vi "Autonomous Independent.vi"() -> ()   [LabVIEW 2011]
doc: "This VI is called when autonomous begins, and will automatically be terminated when autonomous ends. You can carry out timed or sensor driven robot movement independently without needing to return to the caller."
uses:
  <vilib>/Rock Robotics/WPI/Relay/WPI_RelayValue.ctl
  Robot Global Data.vi
  <vilib>/Rock Robotics/WPI/RobotDrive/WPI_RobotDriveArcadeDrive_Standard(NoSaturation).vi
  cupStateGlobal.vi
  InfoTransferGlobal.vi
  <vilib>/ptbypt/NI_PtbyPt.lvlib
panel:
  out "Fixed Distance[m]":dbl
  in  "Slide 3":dbl(slide) scale=400.0..2000.0
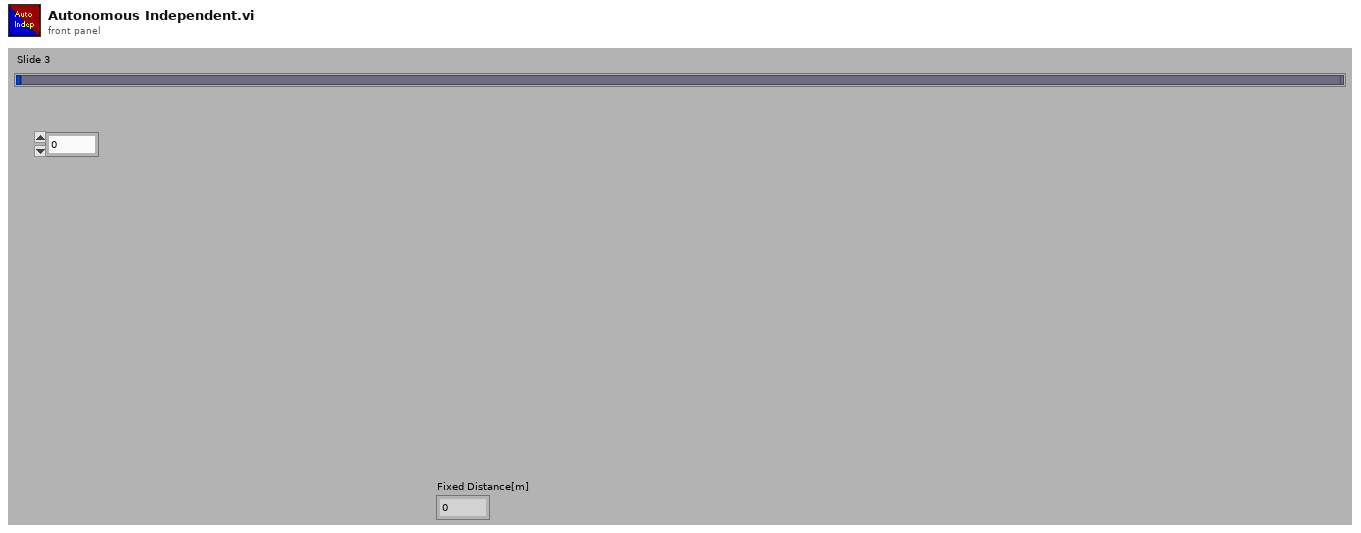
[diagram p1: front panel]
types:
  T1 = typedef "WPI_JoystickDevRef.ctl" = cluster{"Device":T2}
  T2 = typedef "WPI_JoystickDeviceEnum.ctl" = enum16{"USB 1", "USB 2", "USB 3", "USB 4", "Kinect 1", "Kinect 2"}
  T3 = typedef "WPI_DigitalInputDevRef.ctl" = cluster{"DevStatus":errorcluster, "DIO Channel":T4, "Digital Module":T5}
  T4 = typedef "FPGA_DIOChannel.ctl" = enum8{"DIO 1", "DIO 2", "DIO 3", "DIO 4", "DIO 5", "DIO 6", "DIO 7", "DIO 8", "DIO 9", "DIO 10", "DIO 11", "DIO 12", "DIO 13", "DIO 14", "Invalid"}
  T5 = typedef "FPGA_TypedefDigitalModule.ctl" = enum16{"Digital Module 1", "Digital Module 2"}
  T6 = typedef "WPI_RelayValue.ctl" = enum16{"Off", "On", "Forward", "Reverse"}
  T7 = typedef "WPI_RobotDriveDevRef.ctl" = cluster{"DevStatus":errorcluster, "Motors[]":T8[], "Square Inputs":bool, "Max Output":dbl, "Isochronous":bool}
  T8 = typedef "WPI_MotorControlDeviceRef.ctl" = cluster{"DeviceStatus":errorcluster, "Type":enum16{"PWM", "CAN"}, "PWM":cluster{"Digital Module":T5, "PWM Channel":T9, "DeadBand":T10}, "CAN":cluster{"Device Number":u8, "Control Mode":T11, "Semaphore":T12, "Max Vout":dbl}, "Invert":bool, "TransformRef":T13, "InvTransformRef":T13}
  T9 = typedef "FPGA_DIOPWMChannel.ctl" = enum8{"PWM 1", "PWM 2", "PWM 3", "PWM 4", "PWM 5", "PWM 6", "PWM 7", "PWM 8", "PWM 9", "PWM 10", "Invalid"}
  T10 = typedef "WPI_PWMDeadband.ctl" = cluster{"Name":string, "maxPositivePwm":i32, "minPositivePwm":i32, "centerPwm":i32, "maxNegativePwm":i32, "minNegativePwm":i32, "angularRange":u16}
  T11 = typedef "WPI_CANJaguar_ControlMode.ctl" = enum8{"Percent VBus", "Current", "Speed", "Position", "Voltage"}
  T12 = typedef "Semaphore RefNum" = refnum<k1>
  T13 = typedef "WPI_PWMTransform_ConPane.ctl" = refnum<vi>
  T14 = typedef "WPI_EncoderDevRef.ctl" = cluster{"DevStatus":errorcluster, "EncoderIndex":T15, "CounterIndex":T16, "DistancePerCount":dbl, "Decoding Type":T17}
  T15 = typedef "FPGA_EncoderIdx.ctl" = enum8{"Enc 0", "Enc 1", "Enc 2", "Enc 3", "Invalid"}
  T16 = typedef "FPGA_CounterCtrSystemIndex.ctl" = enum8{"Ctr 0", "Ctr 1", "Ctr 2", "Ctr 3", "Ctr 4", "Ctr 5", "Ctr 6", "Ctr 7", "Invalid"}
  T17 = typedef "WPI_EncoderType.ctl" = enum16{"1x", "2x", "4x"}
  T18 = cluster{"RightAxis":dbl, "LeftAxis":dbl, "RightHead":bool, "Left Head":bool, "Left Leg Out":bool, "Left Leg Forward":bool, "Left Leg Back":bool, "Right Leg Out":bool, "Right Leg Forward":bool, "Right Leg Back":bool}
  T19 = typedef "WPI_RelayDevRef.ctl" = cluster{"DevStatus":errorcluster, "Relay Channel":T20, "Digital Module":T5, "Relay Direction":T21}
  T20 = typedef "FPGA_DIORelayChannel.ctl" = enum8{"Relay 1", "Relay 2", "Relay 3", "Relay 4", "Relay 5", "Relay 6", "Relay 7", "Relay 8", "Invalid"}
  T21 = typedef "WPI_RelayDirection.ctl" = enum16{"Both directions", "Forward only", "Reverse only"}
  T22 = typedef "WPI_AnalogChannelDevRef.ctl" = cluster{"DevStatus":errorcluster, "Analog Module":T23, "Analog Channel":T24}
  T23 = typedef "FPGA_TypedefAnalogModule.ctl" = enum16{"Analog Module 1", "Analog Module 2"}
  T24 = typedef "FPGA_AIChannel.ctl" = enum8{"AI 1", "AI 2", "AI 3", "AI 4", "AI 5", "AI 6", "AI 7", "AI 8", "Invalid"}
  T25 = cluster{"Selected Target Info":cluster{"Position":cluster{"X":dbl, "Y":dbl}, "Distance (m)":dbl, "Target Found?":bool}, "output cluster":cluster{"BottomOR":i16, "CupOR":i16, "TopOR":i16, "FloorOR":i16}, "keys pressed":enum16{"0", "1", "2", "3", "4", "5", "6", "7", "8", "9", "A", "B", "C", "D", "E", "F", "G", "H", "I", "J", "K", "L", "M", "N", "O", "P", "Q", "R", "S", "T", "U", "V", "W", "X", "Y", "Z", "F1", "F2", "F3", "F4", "F5", "F6", "F7", "F8", "F9", "F10", "F11", "F12", "F13", "F14", "F15", "ADD", "BACK", "BACKSLASH", "CAPITAL", "COMMA", "DECIMAL", "DELETE", "DIVIDE", "DOWN", "END", "EQUALS", "ESCAPE", "GRAVE (`)", "HOME", "INSERT", "LBRACKET", "LCONTROL", "LEFT", "L ALT", "LSHIFT", "LWIN", "MINUS", "MULTIPLY", "NEXT", "NUMLOCK", "NUMPAD_0", "NUMPAD_1", "NUMPAD_2", "NUMPAD_3", "NUMPAD_4", "NUMPAD_5", "NUMPAD_6", "NUMPAD_7", "NUMPAD_8", "NUMPAD_9", "PAUSE", "PERIOD", "PRIOR (PG UP)", "RBRACKET", "RCONTROL", "RETURN", "RIGHT", "R ALT", "RSHIFT", "RWIN", "SCROLL", "SEMICOLON", "SLASH", "SPACE", "SUBTRACT", "TAB", "UP", "ENTER (num pad)", "' (quote)"}[]}
  T26 = cluster{"Position":cluster{"X":dbl, "Y":dbl}, "Distance (m)":dbl, "Target Found?":bool}
  T27 = typedef "WPI_ServoDeviceRef.ctl" = cluster{"DeviceStatus":errorcluster, "Digital Module":T5, "PWM Channel":T9, "DeadBand":T10}
  T28 = cluster{"axis 1 (x)":dbl, "axis 2 (y)":dbl, "axis 3 (throttle)":dbl, "axis 4":dbl, "axis 5":dbl, "axis 6":dbl}
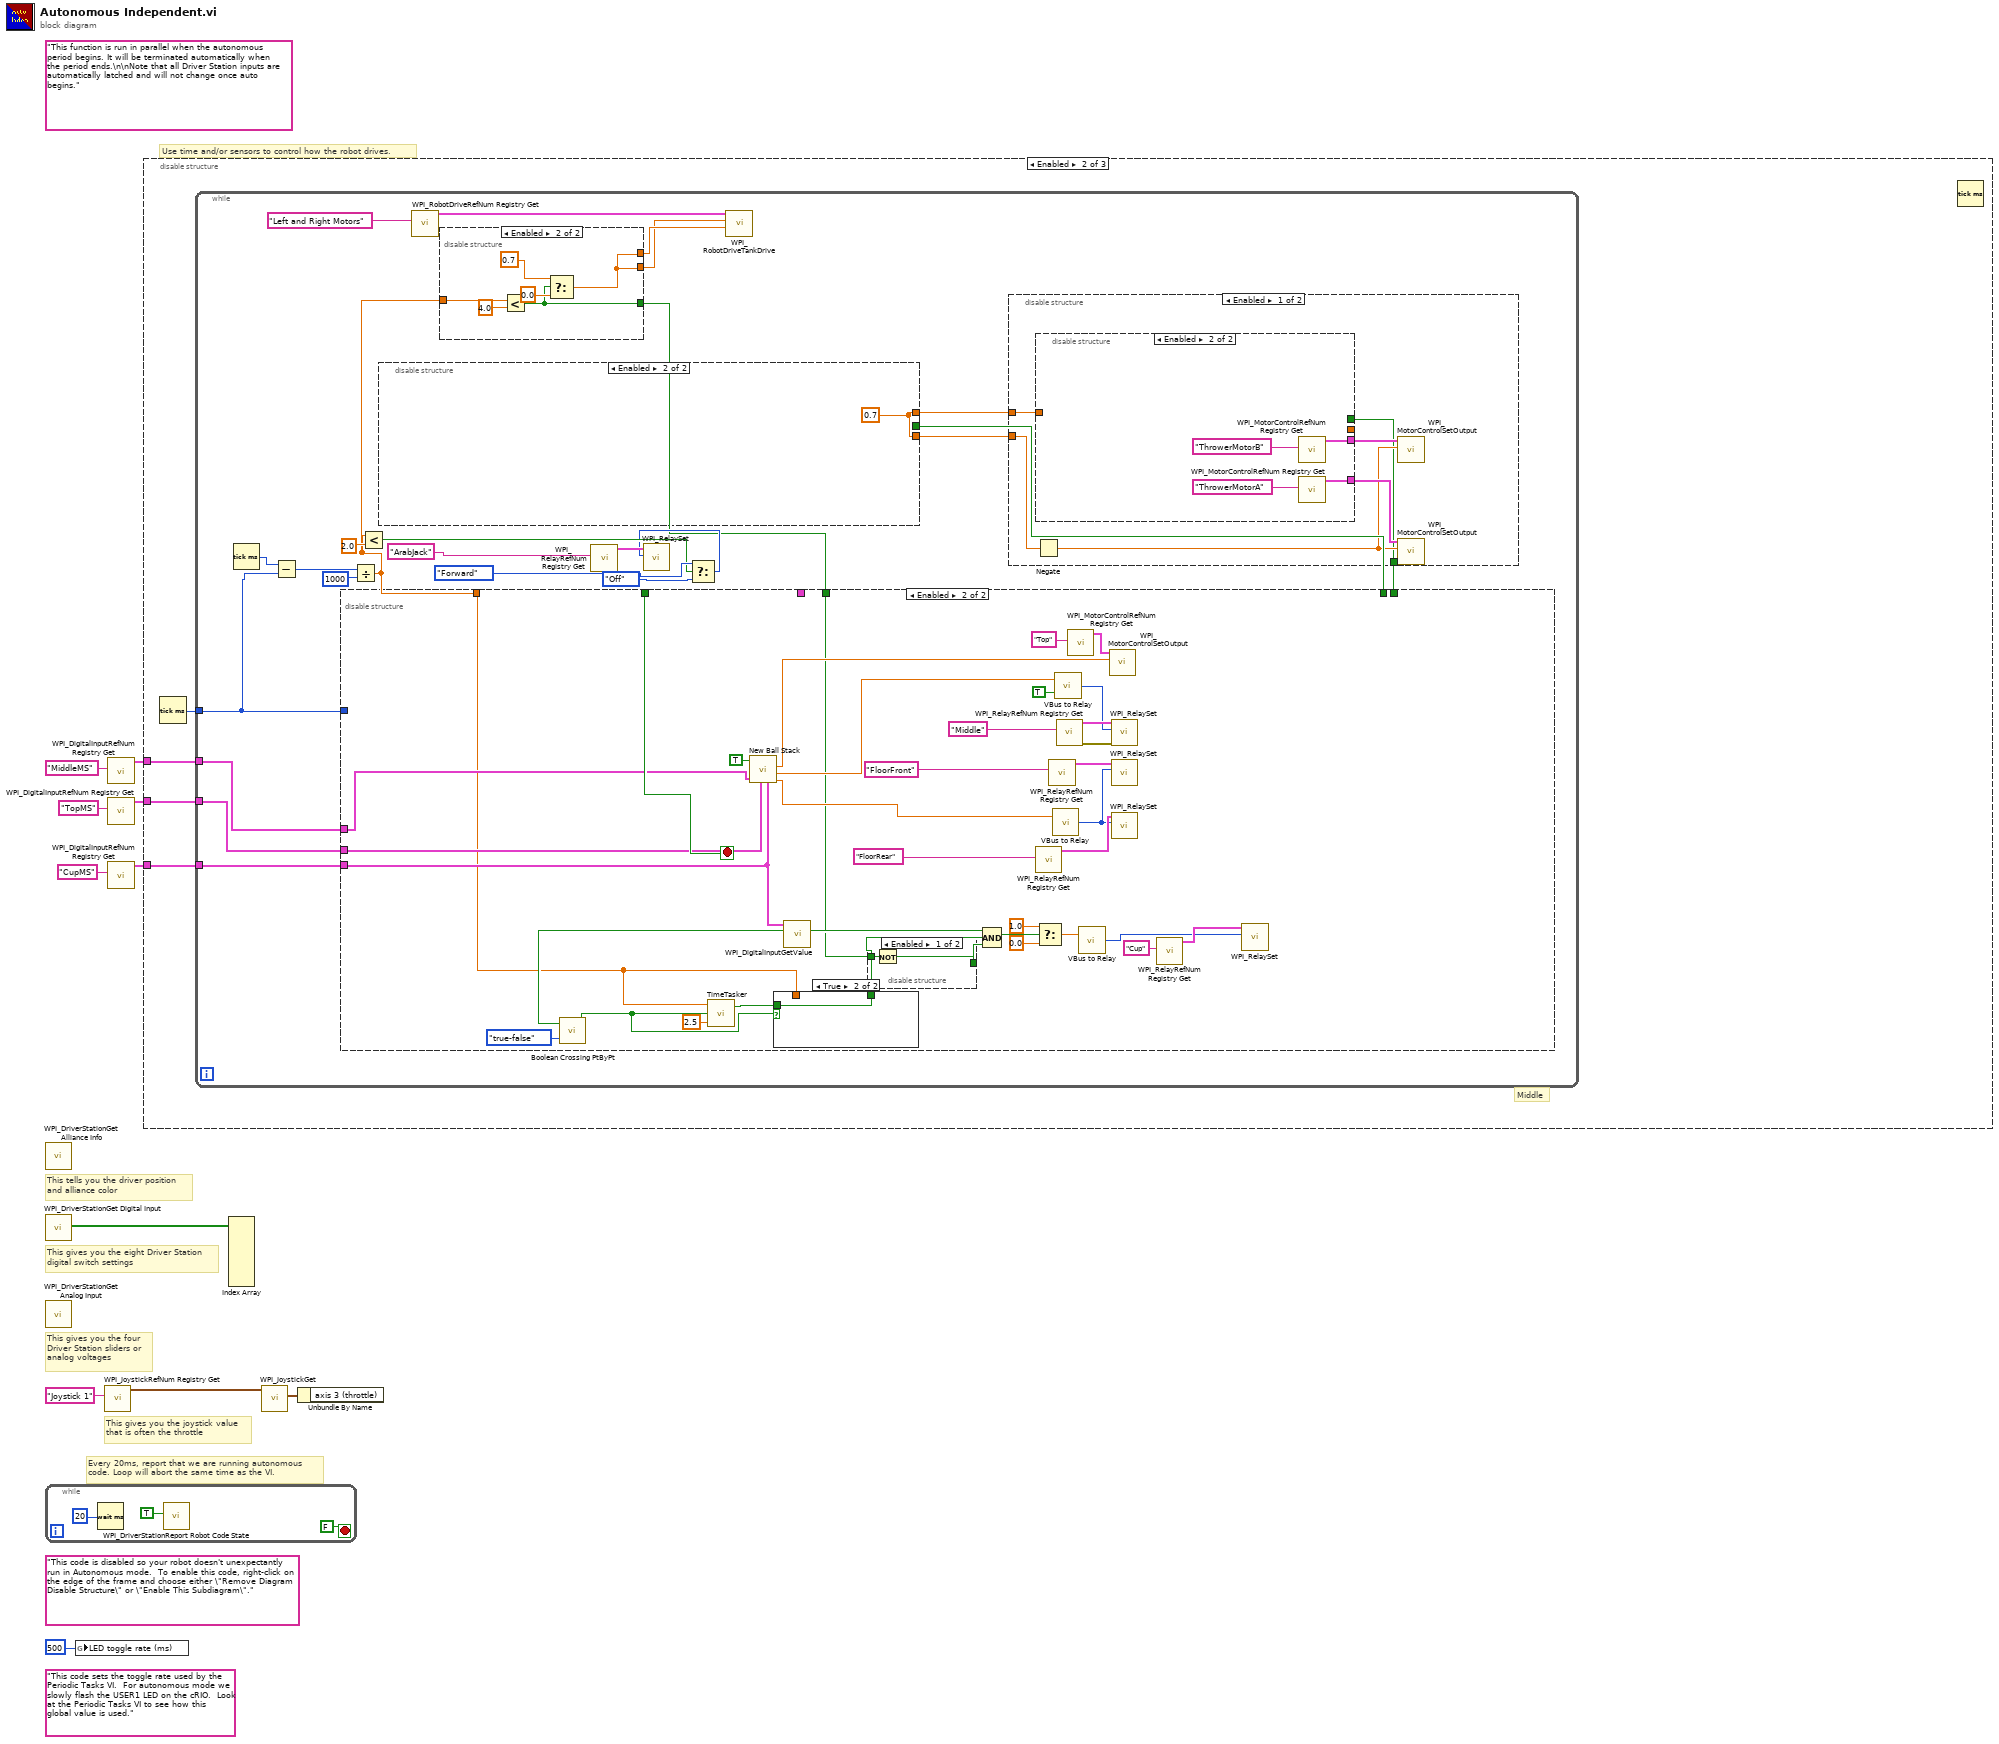
[diagram p0: block diagram]
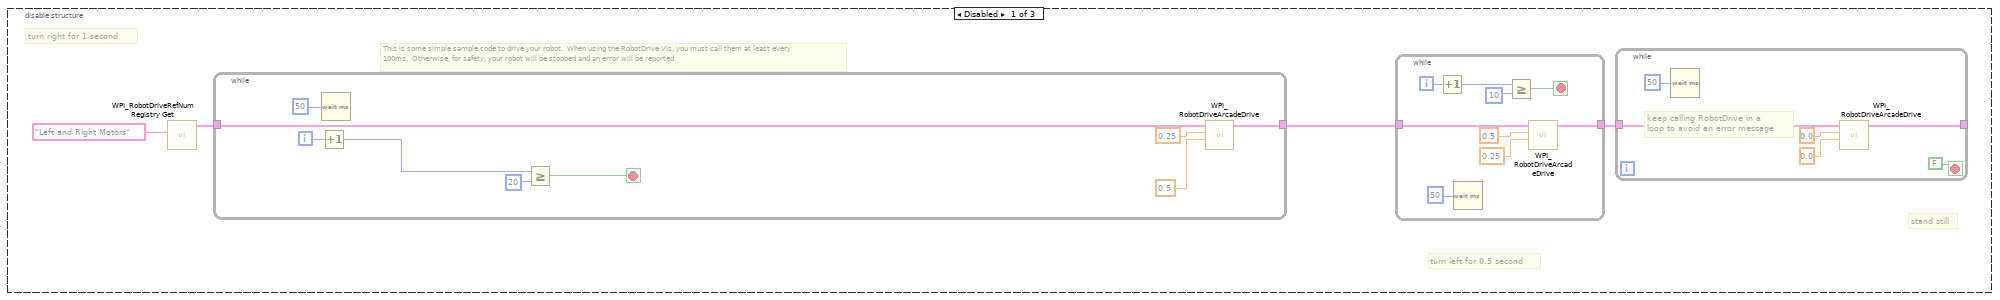
[diagram p2: hidden frame]
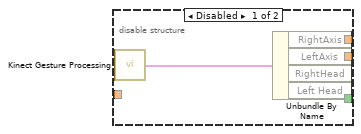
[diagram p3: hidden frame]
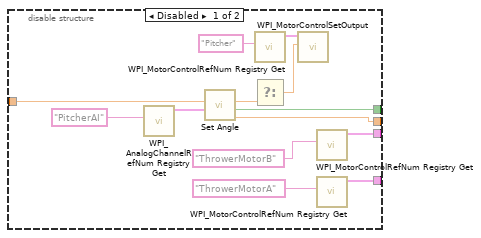
[diagram p4: hidden frame]
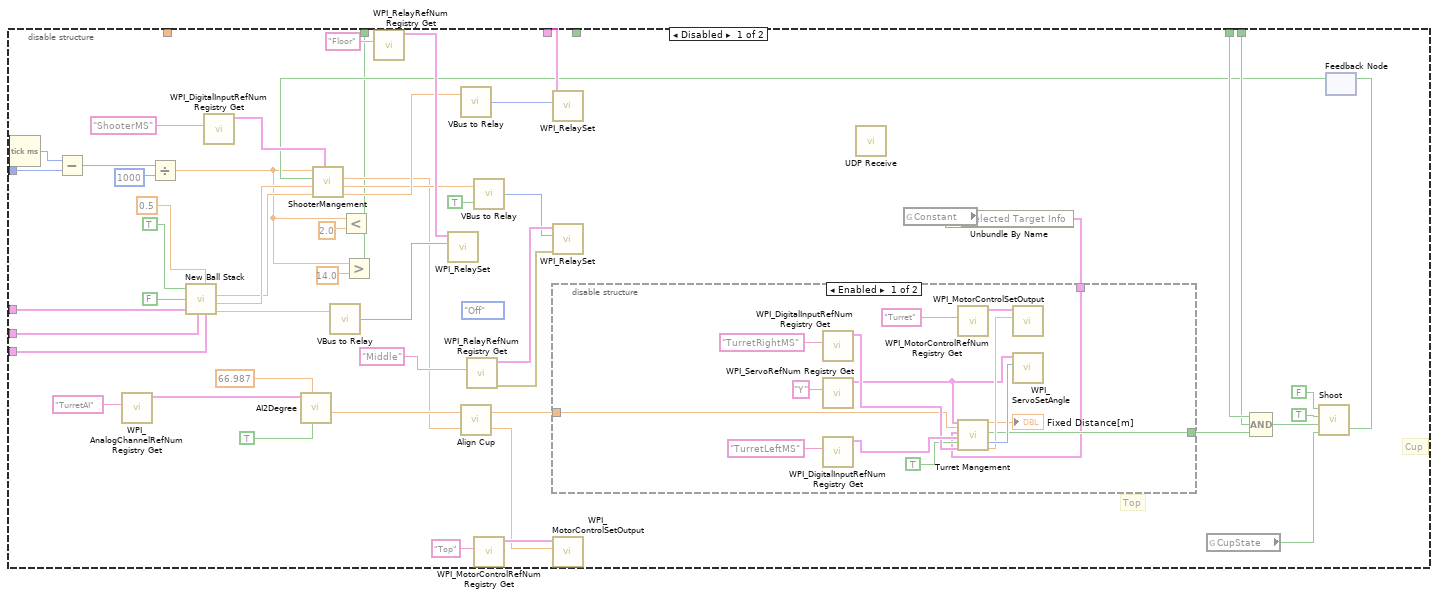
[diagram p6: hidden frame]
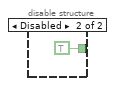
[diagram p8: hidden frame]
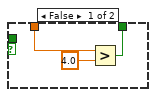
[diagram p9: hidden frame]
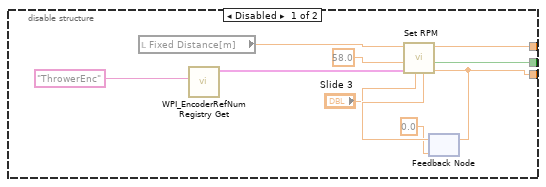
[diagram p10: hidden frame]
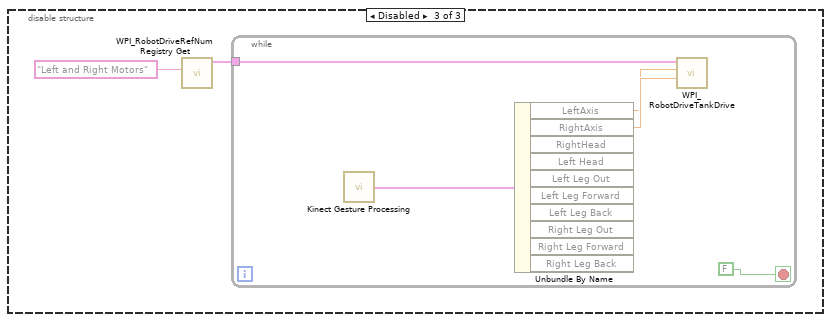
[diagram p11: hidden frame]
diagram:
  (unwired) "This code sets the toggle rate used by the Periodic Tasks VI.  For autonomous mode we slowly flash the USER1 LED on the cRIO.  Look at the Periodic Tasks VI to see how this global value is used."
  (unwired) "This code is disabled so your robot doesn't unexpectantly run in Autonomous mode.  To enable this code, right-click on the edge of the frame and choose either \"Remove Diagram Disable Structure\" or \"Enable This Subdiagram\"."
  (unwired) "This function is run in parallel when the autonomous period begins. It will be terminated automatically when the period ends.\n\nNote that all Driver Station inputs are automatically latched and will not change once auto begins."
  # "Every 20ms, report that we are running autonomous\ncode. Loop will abort the same time as the VI."
  # "This gives you the joystick value\nthat is often the throttle"
  # "Use time and/or sensors to control how the robot drives."
  # "This tells you the driver position\nand alliance color"
  # "This gives you the eight Driver Station\ndigital switch settings"
  # "This gives you the four\nDriver Station sliders or\nanalog voltages"
  n1 = call <vilib>:"WPI_DriverStationGet Alliance Info.vi"() -> ()  [unwired: 12 out]
  n2 = call <vilib>:"WPI_DriverStationGet Digital Input.vi"() -> ("Driver Station Digital Input (1-8)"=w11:bool[])  [unwired: 11 out]
  n3 = call <vilib>:"WPI_DriverStationGet Analog Input.vi"() -> ()  [unwired: 12 out]
  n4 = while {
    stop <- FALSE stop-if-true
    n5 = Wait (ms)(milliseconds to wait=u32 20) -> ()  [unwired: 1 out]
    n6 = call <vilib>:"WPI_DriverStationReport Robot Code State.vi"("Autonomous"=TRUE) -> ()  [unwired: 10 in, 1 out]
  }
  n7 = global write "Robot Global Data.vi" "LED toggle rate (ms)"(u32 500 ("LED ms toggle rate")) -> ()
  n8 = call <vilib>:"WPI_JoystickRefNum Registry Get.vi"("refnum name"="Joystick 1") -> ("JoystickDevRef"=w8:T1)  [unwired: 1 in, 9 out]
  n9 = call <vilib>:"WPI_DigitalInputRefNum Registry Get.vi"("refnum name"="MiddleMS") -> ("DigitalInputDevRef"=w1:T3)  [unwired: 9 in, 1 out]
  n10 = call <vilib>:"WPI_DigitalInputRefNum Registry Get.vi"("refnum name"="TopMS") -> ("DigitalInputDevRef"=w2:T3)  [unwired: 9 in, 1 out]
  n11 = call <vilib>:"WPI_DigitalInputRefNum Registry Get.vi"("refnum name"="CupMS") -> ("DigitalInputDevRef"=w3:T3)  [unwired: 9 in, 1 out]
  n12 = disable-structure shown="Enabled" {
    disable-tunnel: w3 -> [_ w45 _]
    disable-tunnel: w2 -> [_ w46 _]
    disable-tunnel: w1 -> [_ w44 _]
    frame Disabled {
      # "This is some simple sample code to drive your robot.  When using the RobotDrive VIs, you must call them at least every 100ms.  Otherwise, for safety, your robot will be stopped and an error will be reported."
      # "stand still"
      # "turn left for 0.5 second"
      # "turn right for 1 second"
      n13 = call <vilib>:"WPI_RobotDriveRefNum Registry Get.vi"("refnum name"="Left and Right Motors") -> ("RobotDriveDevRef"=w17:T7)  [unwired: 1 in, 9 out]
      n14 = while {
        tunnel: w17 -> [w42]
        tunnel: [w35] -> w16
        i -> [w38]
        stop <- w36 stop-if-true
        n15 = Increment(x=w38) -> (x+1=w34:i32)
        n16 = Wait (ms)(milliseconds to wait=u32 50) -> ()  [unwired: 1 out]
        n17 = Greater Or Equal?(x=w34, y=20) -> (x >= y?=w36:bool)
        n18 = call-poly <vilib>:"WPI_RobotDriveArcadeDrive.vi"("Y axis value"=0.5 ("X axis value"), "X axis value"=0.25, "RobotDriveDevRef"=w42) -> ("RobotDriveDevRef"=w35:T7)  [unwired: 1 in, 7 out]
      }
      n19 = while {
        tunnel: w16 -> [w33]
        tunnel: [w26] -> w15
        i -> [w29]
        stop <- w27 stop-if-true
        n20 = Increment(x=w29) -> (x+1=w25:i32)
        n21 = Wait (ms)(milliseconds to wait=u32 50) -> ()  [unwired: 1 out]
        n22 = Greater Or Equal?(x=w25, y=10) -> (x >= y?=w27:bool)
        n23 = call-poly <vilib>:"WPI_RobotDriveArcadeDrive.vi"("Y axis value"=0.25 ("X axis value"), "X axis value"=0.5, "RobotDriveDevRef"=w33) -> ("RobotDriveDevRef"=w26:T7)  [unwired: 1 in, 7 out]
      }
      n24 = while {
        tunnel: w15 -> [w24]
        tunnel: [w20] -> _
        stop <- FALSE stop-if-true
        # "keep calling RobotDrive in a loop to avoid an error message"
        n25 = Wait (ms)(milliseconds to wait=u32 50) -> ()  [unwired: 1 out]
        n26 = call-poly <vilib>:"WPI_RobotDriveArcadeDrive.vi"("Y axis value"=0.0 ("X axis value"), "X axis value"=0.0, "RobotDriveDevRef"=w24) -> ("RobotDriveDevRef"=w20:T7)  [unwired: 1 in, 7 out]
      }
    }
    frame Enabled {
      # "Middle"
      n27 = Tick Count (ms)() -> (millisecond timer value=w43:u32)
      n28 = while {
        tunnel: w46 -> [w69]
        tunnel: w45 -> [w68]
        tunnel: w44 -> [w67]
        tunnel: w43 -> [w56]
        stop <- w64 stop-if-true
        n29 = Tick Count (ms)() -> (millisecond timer value=w59:u32)
        n30 = Subtract(x=w59, y=w56) -> (x-y=w58:u32)
        n31 = Divide(x=w58, y=u32 1000 ("milliseconds to wait")) -> (x/y=w48:dbl)
        n32 = Less?(x=w48, y=2.0) -> (x < y?=w51:bool)
        n33 = disable-structure shown="Enabled" {
          disable-tunnel: [w224 _] -> w66
          disable-tunnel: [w219 w225] -> w71
          disable-tunnel: [w218 w225] -> w70
          frame Disabled {
            n34 = local read "Fixed Distance[m]"() -> (w215:dbl)
            n35 = call <vilib>:"WPI_EncoderRefNum Registry Get.vi"("refnum name"="ThrowerEnc") -> ("EncoderDevRef"=w223:T14)  [unwired: 9 in, 1 out]
            n36 = feedback #1(0.0 ("Thrower Voltage")) -> (w221:dbl)
            n37 = call "Set RPM.vi"("Last Thrower Voltage (node)"=w221, "Position"="Slide 3", "EncoderDevRef"=w223, "Height"=58.0 ("Angle"), "Distance"=w215) -> ("Thrower Voltage"=w218:dbl, "RPM SET"=w224:bool, "angle"=w219:dbl)  [unwired: 4 in]
            n38 = feedback-in #1(w218) -> ()
          }
          frame Enabled {
            w225 = 0.7 ("MotorPower 3")
          }
        }
        n39 = call <vilib>:"WPI_RobotDriveRefNum Registry Get.vi"("refnum name"="Left and Right Motors") -> ("RobotDriveDevRef"=w61:T7)  [unwired: 9 in, 1 out]
        n40 = disable-structure shown="Enabled" {
          disable-tunnel: [w73 w76] -> w63
          disable-tunnel: [w72 w76] -> w62
          disable-tunnel: w48 -> [_ w80]
          disable-tunnel: [_ w75] -> w47
          frame Disabled {
            n41 = call "Kinect Gesture Processing.vi"() -> ("Joystick Data"=w74:T18)  [unwired: 1 in]
            n42 = Unbundle By Name(w74) -> ("RightAxis"=w73:dbl, "LeftAxis"=w72:dbl)  [unwired: 2 out]
          }
          frame Enabled {
            n43 = Less?(x=w80, y=4.0) -> (x < y?=w75:bool)
            n44 = Select(t=0.7 ("RightAxis"), s=w75, f=0.0) -> (s? t:f=w76:dbl)
          }
        }
        n45 = call <vilib>:"WPI_RelayRefNum Registry Get.vi"("refnum name"="ArabJack") -> ("RelayDevRef"=w54:T19)  [unwired: 9 in, 1 out]
        n46 = Select(t=WPI_RelayValue."Forward" ("RelayValue"), s=w51, f=WPI_RelayValue."Off" ("RelayValue")) -> (s? t:f=w49:T6)
        n47 = call <vilib>:"WPI_RelaySet.vi"("RelayValue"=w49, "RelayDevRef"=w54) -> ()  [unwired: 8 in, 2 out]
        n48 = call <vilib>:"WPI_RobotDriveTankDrive.vi"("Right axis value"=w63, "Left axis value"=w62, "RobotDriveDevRef"=w61) -> ()  [unwired: 7 in, 2 out]
        n49 = disable-structure shown="Enabled" {
          disable-tunnel: w71 -> [w86 _]
          disable-tunnel: w70 -> [w83 _]
          disable-tunnel: [w81 _] -> w65
          frame Enabled {
            n50 = Negate(x=w83) -> (-x=w82:dbl)
            n51 = disable-structure shown="Enabled" {
              disable-tunnel: [w99 _] -> w81
              disable-tunnel: w86 -> [w87 _]
              disable-tunnel: [w96 w101] -> w85
              disable-tunnel: [w95 w100] -> w84
              disable-tunnel: [w90 _] -> _
              frame Disabled {
                n52 = call <vilib>:"WPI_AnalogChannelRefNum Registry Get.vi"("refnum name"="PitcherAI") -> ("AIDeviceRef"=w92:T22)  [unwired: 9 in, 1 out]
                n53 = call "Set Angle.vi"("AIDeviceRef"=w92, "Angle"=w87) -> ("Current Angle(above Horizon)"=w90:dbl, "Angle SET"=w99:bool, "Angle Motor"=w88:dbl)  [unwired: 7 in]
                n54 = call <vilib>:"WPI_MotorControlRefNum Registry Get.vi"("refnum name"="Pitcher") -> ("MotorControlDevRef"=w91:T8)  [unwired: 9 in, 1 out]
                n55 = Select(f=w88) -> (s? t:f=w89:dbl)  [unwired: 2 in]
                n56 = call <vilib>:"WPI_MotorControlSetOutput.vi"("Output"=w89, "MotorControlDevRef"=w91) -> ()  [unwired: 8 in, 2 out]
                n57 = call <vilib>:"WPI_MotorControlRefNum Registry Get.vi"("refnum name"="ThrowerMotorB") -> ("MotorControlDevRef"=w95:T8)  [unwired: 9 in, 1 out]
                n58 = call <vilib>:"WPI_MotorControlRefNum Registry Get.vi"("refnum name"="ThrowerMotorA") -> ("MotorControlDevRef"=w96:T8)  [unwired: 9 in, 1 out]
              }
              frame Enabled {
                n59 = call <vilib>:"WPI_MotorControlRefNum Registry Get.vi"("refnum name"="ThrowerMotorB") -> ("MotorControlDevRef"=w100:T8)  [unwired: 9 in, 1 out]
                n60 = call <vilib>:"WPI_MotorControlRefNum Registry Get.vi"("refnum name"="ThrowerMotorA") -> ("MotorControlDevRef"=w101:T8)  [unwired: 9 in, 1 out]
              }
            }
            n61 = call <vilib>:"WPI_MotorControlSetOutput.vi"("Output"=w82, "MotorControlDevRef"=w84) -> ()  [unwired: 8 in, 2 out]
            n62 = call <vilib>:"WPI_MotorControlSetOutput.vi"("Output"=w82, "MotorControlDevRef"=w85) -> ()  [unwired: 8 in, 2 out]
          }
          frame Disabled {
          }
        }
        n63 = disable-structure shown="Enabled" {
          disable-tunnel: _ -> [w157 _]
          disable-tunnel: w69 -> [w151 w191]
          disable-tunnel: w68 -> [w150 w186]
          disable-tunnel: w67 -> [w149 w190]
          disable-tunnel: w66 -> [w124 _]
          disable-tunnel: w65 -> [w123 _]
          disable-tunnel: w56 -> [w113 _]
          disable-tunnel: [w110 _] -> w64
          disable-tunnel: w48 -> [_ w177]
          disable-tunnel: w47 -> [_ w173]
          frame Disabled {
            w106 = WPI_RelayValue."Off" ("RelayValue")
            # "Top"
            # "Cup"
            n64 = Tick Count (ms)() -> (millisecond timer value=w112:u32)
            n65 = Subtract(x=w112, y=w113) -> (x-y=w114:u32)
            n66 = call <vilib>:"WPI_AnalogChannelRefNum Registry Get.vi"("refnum name"="TurretAI") -> ("AIDeviceRef"=w133:T22)  [unwired: 9 in, 1 out]
            n67 = Divide(x=w114, y=u32 1000 ("milliseconds to wait")) -> (x/y=w109:dbl)
            n68 = call "New Ball Stack.vi"("Suck?"=TRUE, "spinOut?"=FALSE, "MiddleMS"=w149, "TopMS"=w151, "Top Stack Speed"=0.5, "CupMS"=w150) -> ("Top"=w147:dbl, "Middle"=w148:dbl, "Floor"=w126:dbl)  [unwired: 2 in]
            n69 = call <vilib>:"WPI_DigitalInputRefNum Registry Get.vi"("refnum name"="ShooterMS") -> ("DigitalInputDevRef"=w145:T3)  [unwired: 9 in, 1 out]
            n70 = call "AI2Degree.vi"("Invert"=TRUE, "Calibrate"=66.987 ("y"), "AIDeviceRef"=w133) -> ("Degree"=w131:dbl)  [unwired: 8 in]
            n71 = call "VBus to Relay.vi"("Motor VBus"=w126) -> ("RelayValue"=w130:T6)  [unwired: 1 in]
            n72 = Less?(x=w109, y=2.0) -> (x < y?=w107:bool)
            n73 = Greater?(x=w109, y=14.0) -> (0:w110:bool)
            n74 = call <vilib>:"WPI_RelayRefNum Registry Get.vi"("refnum name"="Floor") -> ("RelayDevRef"=w155:T19)  [unwired: 9 in, 1 out]
            n75 = call <vilib>:"WPI_RelaySet.vi"("RelayValue"=w130, "RelayDevRef"=w155) -> ()  [unwired: 8 in, 2 out]
            n76 = call <vilib>:"WPI_RelayRefNum Registry Get.vi"("refnum name"="Middle") -> ("error out"=w140:errorcluster, "RelayDevRef"=w141:T19)  [unwired: 9 in]
            n77 = call <vilib>:"WPI_MotorControlRefNum Registry Get.vi"("refnum name"="Top") -> ("MotorControlDevRef"=w136:T8)  [unwired: 9 in, 1 out]
            n78 = call "UDP Receive.vi"() -> ()  [unwired: 2 in]
            n79 = global read "InfoTransferGlobal.vi" "Constant"() -> (w105:T25)
            n80 = Unbundle By Name(w105) -> ("Selected Target Info"=w104:T26)
            n81 = global read "cupStateGlobal.vi" "CupState"() -> (w118:bool)
            n82 = feedback #2() -> (w116:bool)  [unwired: 1 in]
            n83 = call "ShooterMangement.vi"("Shooter MS"=w145, "Top"=w147, "Middle"=w148, "Le Shoot"=w116, "TeleOp Elapsed Seconds"=w109) -> ("Cup Gain"=w144:dbl, "Middle"=w137:dbl, "Top"=w127:dbl)  [unwired: 4 in]
            n84 = call "VBus to Relay.vi"("Motor VBus"=w144) -> ("RelayValue"=w143:T6)  [unwired: 1 in]
            n85 = call "Align Cup.vi"("Top Input"=w127, "Turret Angle"=w131) -> ("Top Output"=w129:dbl, "Turret Output"=w125:dbl)
            n86 = call "VBus to Relay.vi"("Invert Relay? (F)"=TRUE, "Motor VBus"=w137) -> ("RelayValue"=w138:T6)
            n87 = call <vilib>:"WPI_RelaySet.vi"("RelayValue"=w143, "RelayDevRef"=w157) -> ()  [unwired: 8 in, 2 out]
            n88 = call <vilib>:"WPI_RelaySet.vi"("error in (no error)"=w140, "RelayValue"=w138, "RelayDevRef"=w141) -> ()  [unwired: 7 in, 2 out]
            n89 = disable-structure shown="Enabled" {
              disable-tunnel: w125 -> [w161 _]
              disable-tunnel: [w160 _] -> w122
              disable-tunnel: w104 -> [w158 _]
              frame Enabled {
                n90 = call <vilib>:"WPI_DigitalInputRefNum Registry Get.vi"("refnum name"="TurretRightMS") -> ("DigitalInputDevRef"=w165:T3)  [unwired: 9 in, 1 out]
                n91 = call <vilib>:"WPI_ServoRefNum Registry Get.vi"("refnum name"="Y") -> ("ServoDeviceRef"=w162:T27)  [unwired: 9 in, 1 out]
                n92 = call <vilib>:"WPI_DigitalInputRefNum Registry Get.vi"("refnum name"="TurretLeftMS") -> ("DigitalInputDevRef"=w166:T3)  [unwired: 9 in, 1 out]
                n93 = call <vilib>:"WPI_MotorControlRefNum Registry Get.vi"("refnum name"="Turret") -> ("MotorControlDevRef"=w168:T8)  [unwired: 9 in, 1 out]
                n94 = call "Turret Mangement.vi"("Servo"=w162, "Straigthener"=w161, "DashBoard Info"=w158, "Left"=w166, "AutoSearch"=TRUE ("Sync cam&cannon 4"), "Right"=w165) -> ("Fixed Height[m]"=→"Fixed Distance[m]":dbl, "Locked On Target"=w160:bool, "Servo"=w167:i32, "Turret"=w164:dbl)  [unwired: 8 in, 2 out]
                n95 = call <vilib>:"WPI_MotorControlSetOutput.vi"("Output"=w164, "MotorControlDevRef"=w168) -> ()  [unwired: 8 in, 2 out]
                n96 = call <vilib>:"WPI_ServoSetAngle.vi"("Angle"=w167, "ServoDeviceRef"=w162) -> ()  [unwired: 8 in, 2 out]
              }
              frame Disabled {
              }
            }
            n97 = call <vilib>:"WPI_MotorControlSetOutput.vi"("Output"=w129, "MotorControlDevRef"=w136) -> ()  [unwired: 8 in, 2 out]
            n98 = Compound Arithmetic op=AND(w124, w123, w122) -> (w121:bool)
            n99 = call "Shoot.vi"("Stack Loaded?"=w118, "Ready 2 Shoot?"=w121, "Fire"=TRUE, "Override"=FALSE) -> ("Le Fire at Will?"=w117:bool)  [unwired: 1 out]
            n100 = feedback-in #2(w117) -> ()
          }
          frame Enabled {
            n101 = call "New Ball Stack.vi"("Suck?"=TRUE, "MiddleMS"=w190, "TopMS"=w191, "CupMS"=w186) -> ("Top"=w194:dbl, "Middle"=w193:dbl, "Floor"=w192:dbl)  [unwired: 4 in]
            n102 = call <vilib>:"WPI_DigitalInputGetValue.vi"("DigitalInputDevRef"=w186) -> ("Value"=w180:bool)  [unwired: 8 in, 2 out]
            n103 = call <vilib>:"Boolean Crossing PtByPt.vi"("direction"=enum16{"either", "false-true", "true-false"}."true-false", "input"=w180) -> ("crossing"=w179:bool)  [unwired: 1 in]
            n104 = call "TimeTasker.vi"("Delay(sec)"=2.5, "Start Counting?"=w179, "TeleOp Elapsed Seconds"=w177) -> ("TimePast?"=w176:bool)  [unwired: 1 out]
            n105 = case shown="True" w179 {
              tunnel: [w212 w214] -> w178
              tunnel: w177 -> [w211 _]
              tunnel: w176 -> [_ w214]
              frame False {
                n106 = Greater?(x=w211, y=4.0) -> (0:w212:bool)
              }
              frame True {
              }
            }
            n107 = disable-structure shown="Enabled" {
              disable-tunnel: [w209 TRUE] -> w174
              disable-tunnel: w173 -> [w208 _]
              frame Enabled {
                n108 = Not(x=w208) -> (.not. x?=w209:bool)
              }
              frame Disabled {
              }
            }
            n109 = Compound Arithmetic op=AND(w180, w178, w174) -> (w183:bool)
            n110 = call <vilib>:"WPI_RelayRefNum Registry Get.vi"("refnum name"="FloorRear") -> ("RelayDevRef"=w199:T19)  [unwired: 9 in, 1 out]
            n111 = Select(t=1.0, s=w183, f=0.0) -> (s? t:f=w184:dbl)
            n112 = call <vilib>:"WPI_RelayRefNum Registry Get.vi"("refnum name"="FloorFront") -> ("RelayDevRef"=w202:T19)  [unwired: 9 in, 1 out]
            n113 = call "VBus to Relay.vi"("Motor VBus"=w192) -> ("RelayValue"=w198:T6)  [unwired: 1 in]
            n114 = call "VBus to Relay.vi"("Invert Relay? (F)"=TRUE, "Motor VBus"=w193) -> ("RelayValue"=w203:T6)
            n115 = call <vilib>:"WPI_RelayRefNum Registry Get.vi"("refnum name"="Middle") -> ("error out"=w205:errorcluster, "RelayDevRef"=w206:T19)  [unwired: 9 in]
            n116 = call <vilib>:"WPI_MotorControlRefNum Registry Get.vi"("refnum name"="Top") -> ("MotorControlDevRef"=w196:T8)  [unwired: 9 in, 1 out]
            n117 = call "VBus to Relay.vi"("Motor VBus"=w184) -> ("RelayValue"=w187:T6)  [unwired: 1 in]
            n118 = call <vilib>:"WPI_MotorControlSetOutput.vi"("Output"=w194, "MotorControlDevRef"=w196) -> ()  [unwired: 8 in, 2 out]
            n119 = call <vilib>:"WPI_RelaySet.vi"("error in (no error)"=w205, "RelayValue"=w203, "RelayDevRef"=w206) -> ()  [unwired: 7 in, 2 out]
            n120 = call <vilib>:"WPI_RelaySet.vi"("RelayValue"=w198, "RelayDevRef"=w202) -> ()  [unwired: 8 in, 2 out]
            n121 = call <vilib>:"WPI_RelaySet.vi"("RelayValue"=w198, "RelayDevRef"=w199) -> ()  [unwired: 8 in, 2 out]
            n122 = call <vilib>:"WPI_RelayRefNum Registry Get.vi"("refnum name"="Cup") -> ("RelayDevRef"=w188:T19)  [unwired: 9 in, 1 out]
            n123 = call <vilib>:"WPI_RelaySet.vi"("RelayValue"=w187, "RelayDevRef"=w188) -> ()  [unwired: 8 in, 2 out]
          }
        }
      }
      n124 = Tick Count (ms)() -> ()  [unwired: 1 out]
    }
    frame Disabled {
      n125 = call <vilib>:"WPI_RobotDriveRefNum Registry Get.vi"("refnum name"="Left and Right Motors") -> ("RobotDriveDevRef"=w226:T7)  [unwired: 1 in, 9 out]
      n126 = while {
        tunnel: w226 -> [w229]
        stop <- FALSE stop-if-true
        n127 = call "Kinect Gesture Processing.vi"() -> ("Joystick Data"=w232:T18)  [unwired: 1 in]
        n128 = Unbundle By Name(w232) -> ("LeftAxis"=w230:dbl, "RightAxis"=w231:dbl)  [unwired: 8 out]
        n129 = call <vilib>:"WPI_RobotDriveTankDrive.vi"("Right axis value"=w231, "Left axis value"=w230, "RobotDriveDevRef"=w229) -> ()  [unwired: 7 in, 2 out]
      }
    }
  }
  n130 = Index Array(array=w11) -> ()  [unwired: 8 in, 8 out]
  n131 = call <vilib>:"WPI_JoystickGet.vi"("JoystickDevRef"=w8) -> ("Axes"=w9:T28)  [unwired: 1 in, 5 out]
  n132 = Unbundle By Name(w9) -> ()  [unwired: 1 out]
